vi "ProbeCardPositioning.vi"(0 "Refnum in":T1, 1 "error in (no error)":errorcluster, 3 "Stop":bool) -> (7 "Refnum out":T1, 8 "error out":errorcluster, 10 "Image Dst Out":T2)   [LabVIEW 2014]
uses:
  <vilib>/userdefined/High Color/VBAIInterface.ctl
  <vilib>/vision/Image Controls.llb/IMAQ Image.ctl
  c_VBAI_SelcectInspection.ctl
  g_Stop.vi
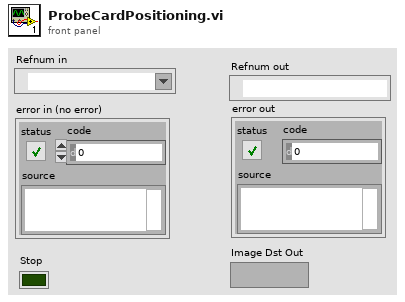
[diagram p1: front panel]
types:
  T1 = typedef "VBAIInterface.ctl" = refnum<k21>
  T2 = typedef "IMAQ Image.ctl" = refnum<image>
  T3 = typedef "c_VBAI_SelcectInspection.ctl" = enum16{"Image Acquisition", "Find Reference", "Chip Alignment", "Adjustment", "Porbecard Positioning"}
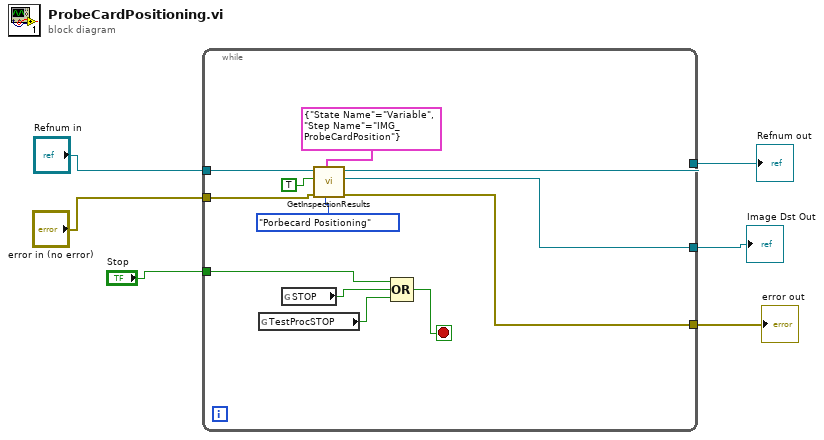
[diagram p0: block diagram]
diagram:
  n1 = while {
    tunnel: [w16] -> w6
    tunnel: "Refnum in" -> [w15]
    tunnel: "error in (no error)" -> [w14]
    tunnel: [w13] -> w3
    tunnel: [w8] -> w2
    tunnel: "Stop" -> [w7]
    stop <- w10 stop-if-true
    n2 = global read "g_Stop.vi" "TestProcSTOP"() -> (w12:bool)
    n3 = global read "g_Stop.vi" "STOP"() -> (w11:bool)
    n4 = call "GetInspectionResults.vi"("Select Inspection"=c_VBAI_SelcectInspection."Porbecard Positioning" ("Enum"), "Image Step Name (default last image used by inspection)"=cluster{"State Name":string, "Step Name":string} {"State Name"="Variable", "Step Name"="IMG_ProbeCardPosition"}, "error in (no error)"=w14, "Image Enable"=TRUE, "Refnum in"=w15) -> ("error out"=w13:errorcluster, "Image Dst Out"=w8:T2, "Refnum out"=w16:T1)  [unwired: 1 in, 3 out]
    n5 = Compound Arithmetic op=OR(w7, w11, w12) -> (w10:bool)
  }
  "Refnum out" <- w6
  "error out" <- w3
  "Image Dst Out" <- w2
